vi "Z6_Beamline_Chief.ProcEvents.vi"(0 "i ref in":refnum<vi>, 5 "error in (no error)":errorcluster) -> (14 "i ref out":refnum<vi>, 19 "error out":errorcluster)   [LabVIEW 2014, in "Z6_Beamline_Chief.lvlib"]
doc: "This method is used to define the events the object will listen to. Add your own events here."
uses:
  Z6_Beamline_Chief.lvlib
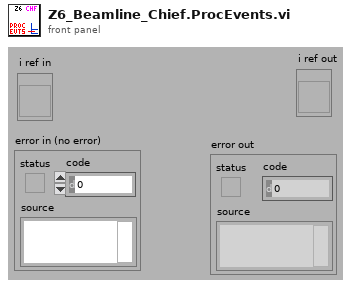
[diagram p1: front panel]
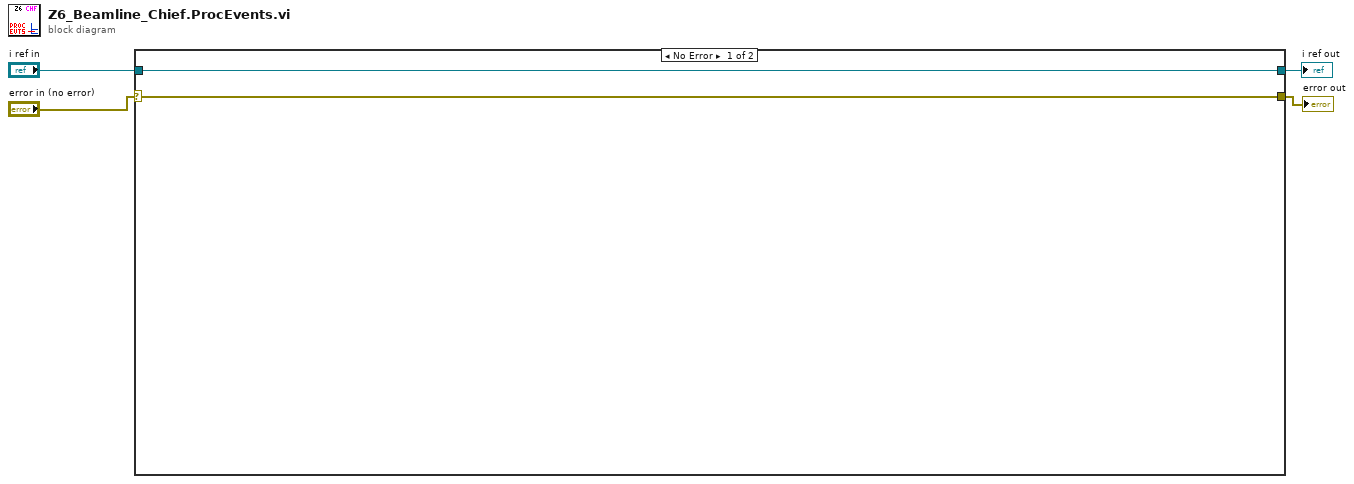
[diagram p0: block diagram]
diagram:
  n1 = case shown="No Error" "error in (no error)" {
    selector: "error in (no error)" -> [w5 w7]
    tunnel: [w5 w7] -> w4
    tunnel: [w6 w8] -> w3
    tunnel: "i ref in" -> [w6 w8]
    frame No Error {
    }
    frame Error {
    }
  }
  "i ref out" <- w3
  "error out" <- w4
